vi "GENser Checksum Append.vi"(8 "error":errorcluster, 10 "Input Cmd":string, 11 "VISA":refnum<visa-resource-name>="COM1") -> (0 "error out":errorcluster, 2 "ChkSum Cmd":string, 3 "VISA out":refnum<visa-resource-name>)   [LabVIEW 2017]
doc: "This vi will add a checksum to any command string.\nThe format of the \"ChkSum Cmd\" output is:\n \"Command\" & \"Dollar Sign\" & \"Two Hex Digits\" & \"Carriage Return\"\n\nThe command is only formulated, it is not sent to the instrument."
panel:
  # "Add Checksum to \n  Command"
  # "Lambda Genesys \n Serial Port\n  DC Power Supplies"
  # "Append \"$xx\" checksum to any\ncommand string if it is not already done"
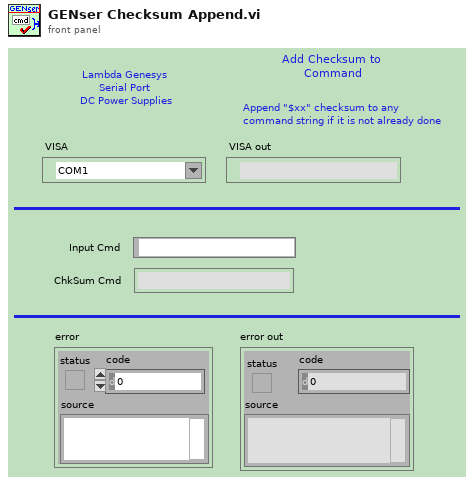
[diagram p1: front panel]
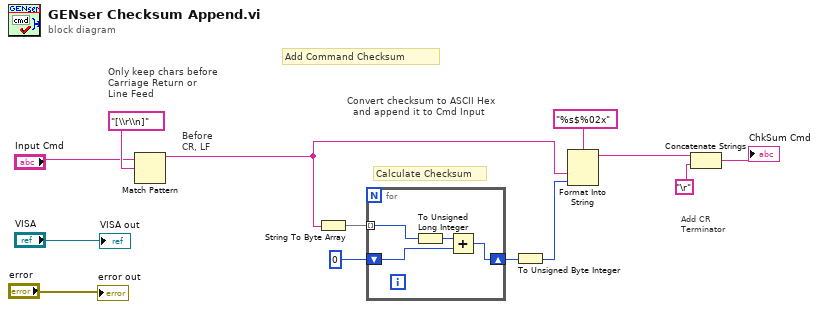
[diagram p0: block diagram]
diagram:
  # "Convert checksum to ASCII Hex  \n  and append it to Cmd Input"
  # "Calculate Checksum"
  # "Add Command Checksum"
  # "Add CR\nTerminator"
  # "Before\nCR, LF"
  # "Only keep chars before\nCarriage Return or\nLine Feed"
  n1 = Match Pattern(string="Input Cmd", regular expression="[\\r\\n]") -> (before substring=w8:string)  [unwired: 1 in, 3 out]
  n2 = String To Byte Array(string=w8) -> (unsigned byte array=w6:u8[])
  n3 = for {
    tunnel: w6 -> [w17] mode=indexing
    shift-right: [w15] -> w4
    shift-left: u32 0 -> [w16]
    n4 = To Unsigned Long Integer(number=w17) -> (unsigned 32bit integer=w14:u32)
    n5 = Add(x=w14, y=w16) -> (x+y=w15:u32)
  }
  n6 = To Unsigned Byte Integer(number=w4) -> (unsigned 8bit integer=w2:u8)
  n7 = Format Into String(format string="%s$%02x" ("regular expression"), w8, w2) -> (resulting string=w9:string)  [unwired: 2 in, 1 out]
  n8 = Concatenate Strings(w9, "\r") -> (→"ChkSum Cmd":string)
  "error out" <- "error"
  "VISA out" <- "VISA"
